vi "TCPReadDBL.vi"(8 "error in (no error)":errorcluster, 9 "timeout ms (25000)":i32, 10 "command":string, 11 "connection ID":refnum<k5>) -> (0 "error out":errorcluster, 2 "DBL value":dbl, 3 "connection ID out":refnum<k5>)   [LabVIEW 2013]
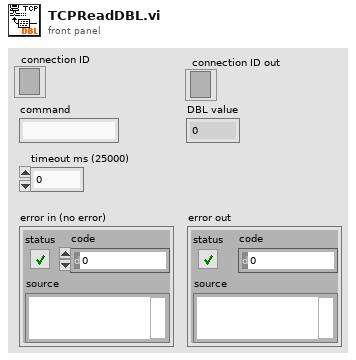
[diagram p1: front panel]
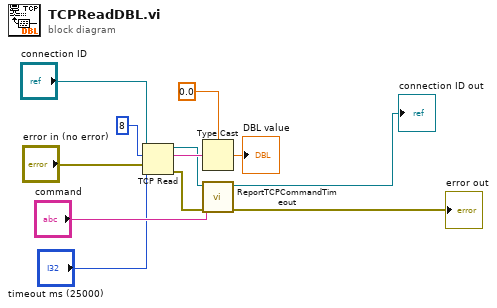
[diagram p0: block diagram]
diagram:
  n1 = TCP Read(connection ID="connection ID", bytes to read=8, error in (no error)="error in (no error)", 9:"timeout ms (25000)") -> (connection ID out=w9:refnum<k5>, data out=w12:string, error out=w10:errorcluster)  [unwired: 1 in]
  n2 = Type Cast(type=0.0 ("DBL value"), x=w12) -> (*(type *) &x=→"DBL value":dbl)
  n3 = call "ReportTCPCommandTimeout.vi"("error in (no error)"=w10, "command"="command", "connection ID"=w9) -> ("error out"=→"error out":errorcluster, "connection ID out"=→"connection ID out":refnum<k5>)  [unwired: 7 in]
